vi "Launch Test Unit.vi"(8 "error in":errorcluster, 9 "Init Module ID":bool, 10 "Number of socket":i32=1 min=1 max=255 step=1, 11 "Message Queue":refnum<class "Delacor_lib_QMH_Message Queue.lvclass">) -> (0 "error out":errorcluster)   [LabVIEW 2025, in "Full User Interface.lvlib"]
uses:
  Full User Interface.lvlib
  <vilib>/Delacor/Delacor QMH/Libraries/Message Queue_class/Delacor_lib_QMH_Message Queue.lvclass
  Test Unit/Test Unit.lvlib
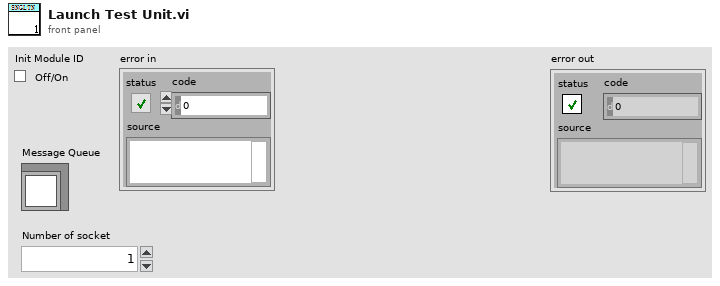
[diagram p1: front panel]
types:
  T1 = typedef "Test Unit.lvlib/Broadcast Events--cluster.ctl" = cluster{"Module Did Init":refnum<user-event>, "Status Updated":refnum<user-event>, "Error Reported":refnum<user-event>, "Module Did Stop":refnum<user-event>, "Update Module Execution Status":refnum<user-event>}
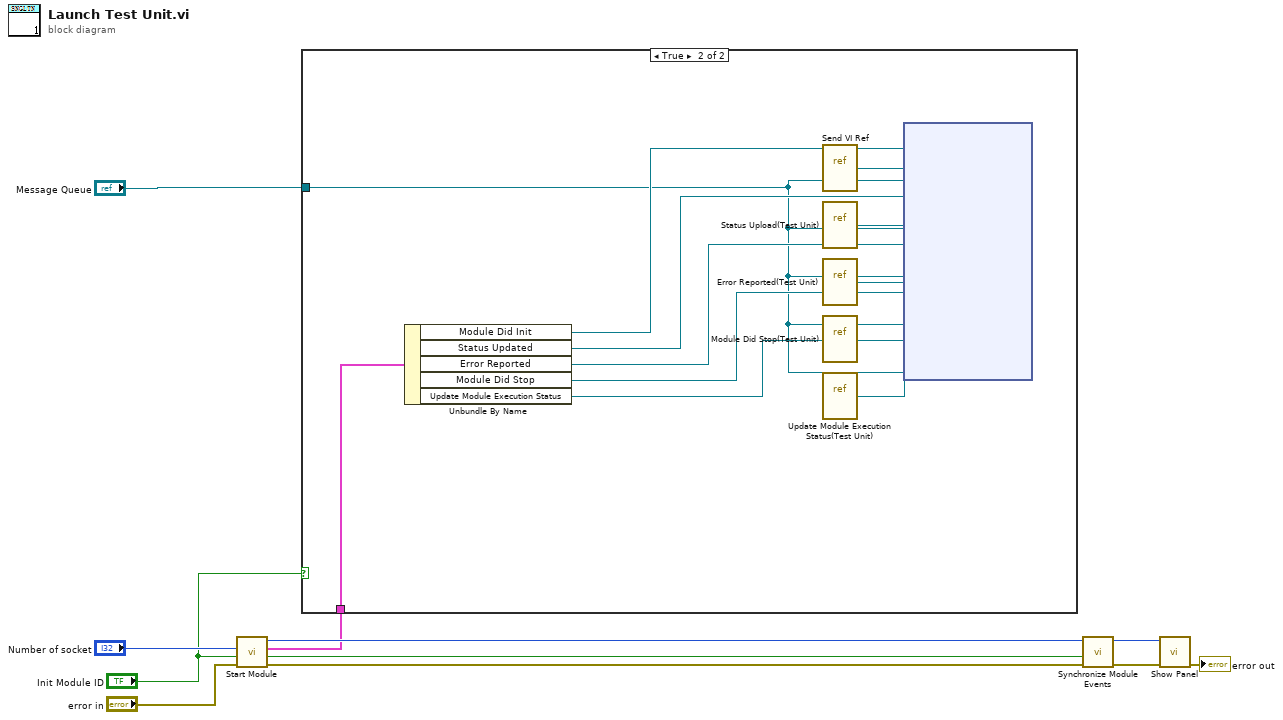
[diagram p0: block diagram]
diagram:
  n1 = call "Start Module.vi"("error in"="error in", "Init Module ID"="Init Module ID", "Number of socket"="Number of socket") -> ("error out"=w4:errorcluster, "Wait for Event Sync?"=w11:bool, "Test Unit Broadcast Events"=w6:T1, "Module ID"=w10:i32)  [unwired: 5 in]
  n2 = case shown="True" "Init Module ID" {
    tunnel: w6 -> [_ w23]
    tunnel: "Message Queue" -> [_ w12]
    frame False {
    }
    frame True {
      n3 = Unbundle By Name(w23) -> ("Module Did Init"=w22:refnum<user-event>, "Status Updated"=w21:refnum<user-event>, "Error Reported"=w20:refnum<user-event>, "Module Did Stop"=w18:refnum<user-event>, "Update Module Execution Status"=w17:refnum<user-event>)
      n4 = vi-ref "Send VI Ref.vi"() -> ("vi reference"=w19:refnum<vi>)
      n5 = vi-ref "Status Upload(Test Unit).vi"() -> ("vi reference"=w16:refnum<vi>)
      n6 = vi-ref "Error Reported(Test Unit).vi"() -> ("vi reference"=w15:refnum<vi>)
      n7 = vi-ref "Module Did Stop(Test Unit).vi"() -> ("vi reference"=w14:refnum<vi>)
      n8 = vi-ref "Update Module Execution Status(Test Unit).vi"() -> ("vi reference"=w13:refnum<vi>)
      n9 = node(w22, w19, w12, w21, w16, w12, w20, w15, w12, w18, w14, w12, w17, w13, w12) -> ()  [unwired: 2 in, 2 out]
    }
  }
  n10 = call "Synchronize Module Events.vi"("error in"=w4, "Wait for Event Sync?"=w11, "Module ID in"=w10) -> ("error out"=w7:errorcluster, "Module ID out"=w8:i32)  [unwired: 7 in]
  n11 = call "Show Panel.vi"("error in"=w7, "Module ID"=w8) -> ("error out"=→"error out":errorcluster)  [unwired: 9 in]
